vi "Multiple Files Handler.vi"(8 "error in (no error)":errorcluster, 11 "TDMS Log":refnum<class "TDMS Logger.lvclass">) -> (0 "error out":errorcluster, 3 "TDMS Log Out":refnum<class "TDMS Logger.lvclass">)   [LabVIEW 2015, in "TDMS Logger.lvlib" / "TDMS Logger.lvclass"]
uses:
  TDMS Logger.lvclass
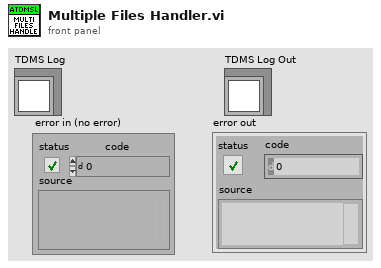
[diagram p1: front panel]
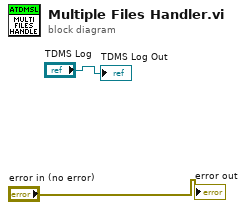
[diagram p0: block diagram]
diagram:
  "TDMS Log Out" <- "TDMS Log"
  "error out" <- "error in (no error)"
